vi "Calculate_(101)_Local_Cost_F()-1.vi"(4 "[IN] Dot matrix with statuses \nfor potentially moving dots":i16[][](array[numeric]), 5 "[IN] Still connected\ntracks in group":T1, 6 "[IN] Potentially\nMoving (X,Y)":dbl[][](array[numeric]), 7 "[IN] Subtracks":T2(array[cluster]), 8 "error IN":errorcluster, 9 "[IN] Areas particles\nPrimary Detected":dbl[][](array[numeric]), 10 "[IN] Primary \n(X,Y) Detected":dbl[][](array[numeric]), 11 "[IN] Cost function":i8[](array[numeric])) -> (0 "error OUT":errorcluster, 3 "[OUT] Cost function":i8[](array[numeric]))   [LabVIEW 2013]
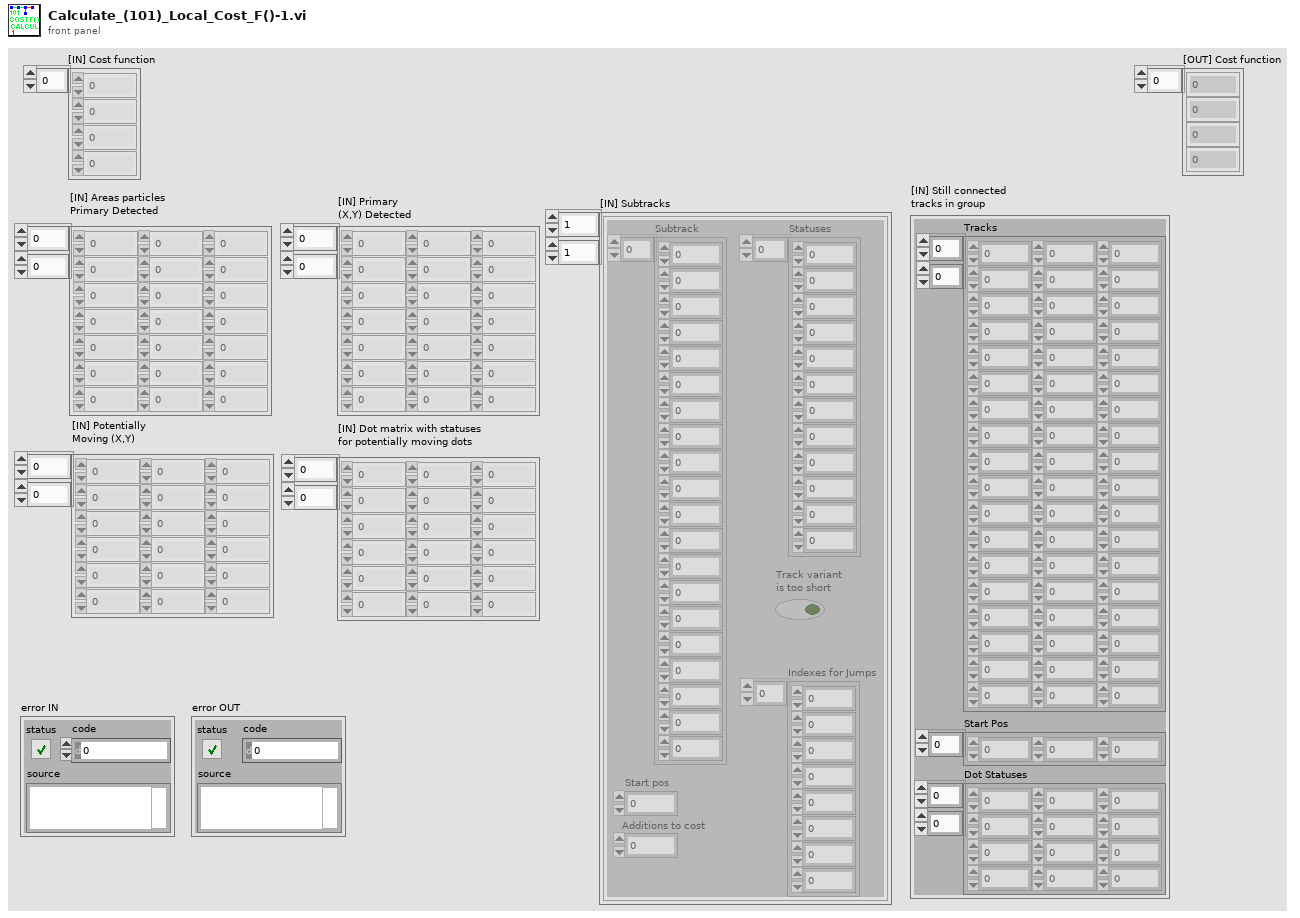
[diagram p1: front panel]
types:
  T1 = cluster{"Tracks":dbl[][], "Start Pos":i32[], "Dot Statuses":i16[][]}
  T2 = cluster{"Subtrack":dbl[], "Statuses":i16[], "Start pos":i32, "Additions to cost":i32, "Track variant \nis too short":bool, "Indexes for Jumps":i32[]}[][]
  T3 = cluster{"Subtrack":dbl[], "Statuses":i16[], "Start pos":i32, "Additions to cost":i32, "Track variant \nis too short":bool, "Indexes for Jumps":i32[]}[]
  T4 = cluster{"Subtrack":dbl[], "Statuses":i16[], "Start pos":i32, "Additions to cost":i32, "Track variant \nis too short":bool, "Indexes for Jumps":i32[]}
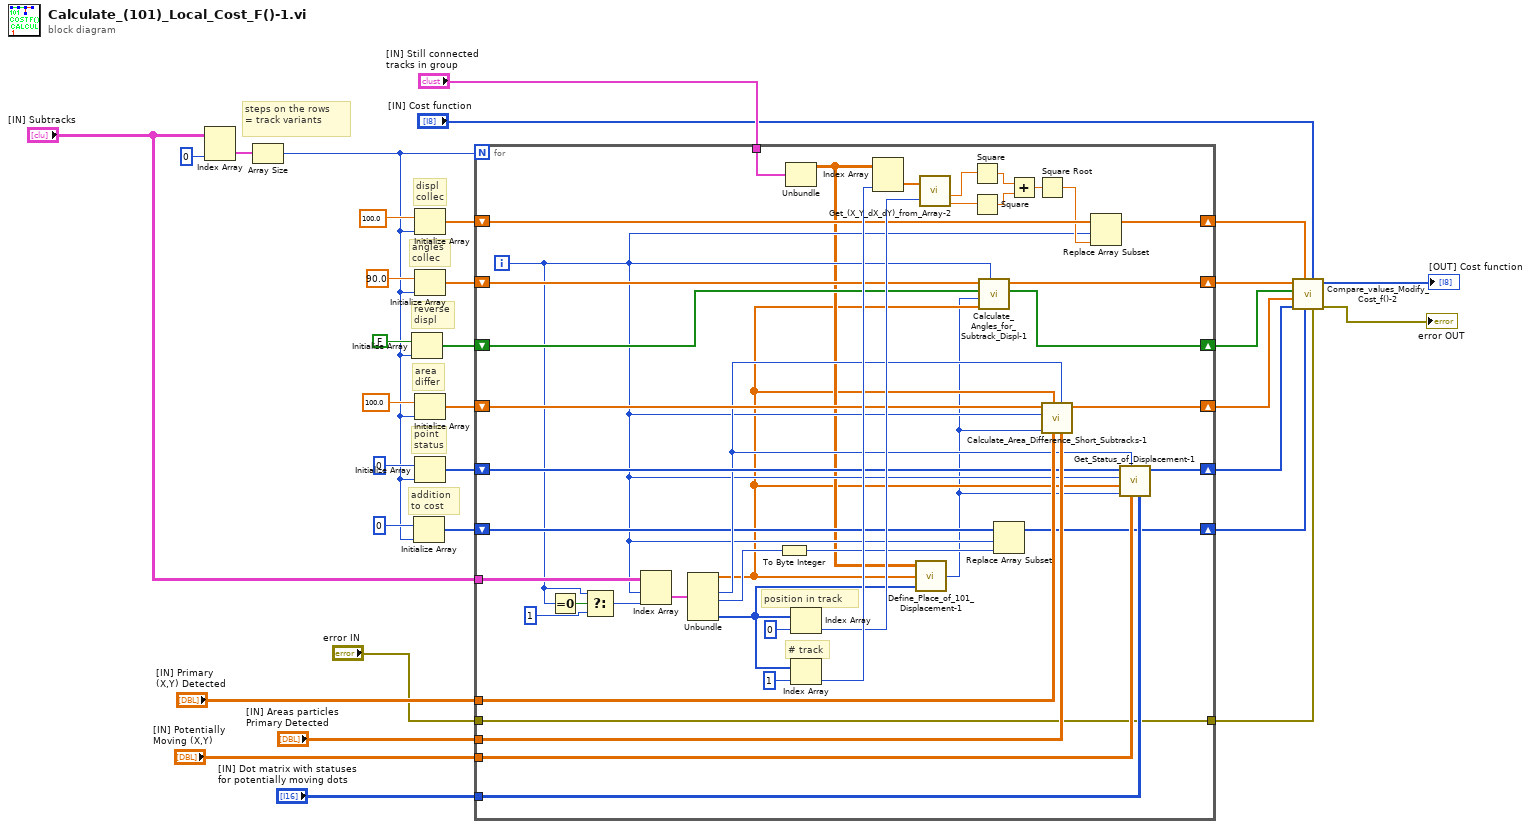
[diagram p0: block diagram]
diagram:
  # "steps on the rows\n= track variants"
  # "addition \nto cost"
  # "point\nstatus"
  # "area \ndiffer"
  # "reverse \ndispl"
  # "angles \ncollec"
  # "displ \ncollec"
  n1 = Index Array(array="[IN] Subtracks", index (col)=0 ("disabled index (col)")) -> (element=w18:T3)  [unwired: 1 in]
  n2 = Array Size(array=w18) -> (size(s)=w17:i32)
  n3 = Initialize Array(FALSE, w17) -> (w27:bool[])
  n4 = Initialize Array(i8 0, w17) -> (w21:i8[])
  n5 = Initialize Array(100.0, w17) -> (w31:dbl[])
  n6 = Initialize Array(90.0, w17) -> (w29:dbl[])
  n7 = Initialize Array(100.0, w17) -> (w25:dbl[])
  n8 = Initialize Array(i16 0, w17) -> (w23:i16[])
  n9 = for {
    N: w17 -> [_]
    tunnel: "[IN] Subtracks" -> [w74]
    tunnel: "[IN] Still connected\ntracks in group" -> [w70]
    shift-right: [w65] -> w6
    shift-left: w31 -> [w66]
    shift-right: [w63] -> w10
    shift-left: w29 -> [w64]
    shift-right: [w61] -> w9
    shift-left: w27 -> [w62]
    tunnel: "[IN] Primary \n(X,Y) Detected" -> [w57]
    tunnel: "[IN] Areas particles\nPrimary Detected" -> [w59]
    shift-right: [w58] -> w8
    shift-left: w25 -> [w60]
    tunnel: "[IN] Potentially\nMoving (X,Y)" -> [w54]
    tunnel: "[IN] Dot matrix with statuses \nfor potentially moving dots" -> [w53]
    shift-right: [w52] -> w7
    shift-left: w23 -> [w56]
    shift-right: [w48] -> w4
    shift-left: w21 -> [w51]
    tunnel: "error IN" -> [w41]
    tunnel: [w41] -> w2
    i -> [w37]
    # "# track"
    # "position in track"
    n10 = Equal To 0?(x=w37) -> (x = 0?=w40:bool)
    n11 = Select(t=w37, s=w40, f=1) -> (s? t:f=w38:i32)
    n12 = Index Array(array=w74, index (row)=w37, index (col)=w38) -> (element=w73:T4)
    n13 = Unbundle(w73) -> ("Subtrack"=w35:dbl[], "Start pos"=w55:i32, "Additions to cost"=w50:i32, "Indexes for Jumps"=w34:i32[])  [unwired: 2 out]
    n14 = To Byte Integer(number=w50) -> (8bit integer=w49:i8)
    n15 = Unbundle(w70) -> ("Tracks"=w36:dbl[][])  [unwired: 2 out]
    n16 = Index Array(array=w34, index=0) -> (element=w67:i32)
    n17 = Index Array(array=w34, index=1) -> (element=w69:i32)
    n18 = Index Array(array=w36, index (col)=w69) -> (element=w68:dbl[])  [unwired: 1 in]
    n19 = call "Define_Place_of_101_Displacement-1.vi"("[IN] Indexes for Jumps"=w34, "[IN] Subtrack"=w35, "[IN] Tracks"=w36) -> ("[OUT] Index of \"11\" Dis\nplacement in Subtrack"=w33:i32)  [unwired: 2 in]
    n20 = call "Get_(X_Y_dX_dY)_from_Array-2.vi"("(X,Y,dX,dY)"=w68, "Index of Displacement"=w67) -> ("dX"=w44:dbl, "dY"=w43:dbl)  [unwired: 2 out]
    n21 = Square(x=w44) -> (x^2=w47:dbl)
    n22 = Square(x=w43) -> (x^2=w46:dbl)
    n23 = call "Calculate_Angles_for_Subtrack_Displ-1.vi"("[IN] Index of subtrack"=w37, "[IN] Subtrack"=w35, "[IN] Index of \"11\" Dis-\nplacement in Subtrack"=w33, "[IN] Reverse Displ or Not"=w62, "[IN] Array with Angles \nBetween Displacement"=w64) -> ("[OUT] Reverse displacement or not"=w61:bool[], "[OUT] Angles betwe\nen two displacements"=w63:dbl[])  [unwired: 3 in]
    n24 = Replace Array Subset(array=w51, new element=w49, index=w37) -> (w48:i8[])
    n25 = Add(x=w47, y=w46) -> (x+y=w45:dbl)
    n26 = Square Root(x=w45) -> (sqrt(x)=w42:dbl)
    n27 = call "Calculate_Area_Difference_Short_Subtracks-1.vi"("[IN] Areas particles\nPrimary Detected"=w59, "[IN] Start pos"=w55, "[IN] Primary \n(X,Y) Detected"=w57, "[IN] Subtrack"=w35, "[IN] Index of \"11\" Dis-\nplacement in Subtrack"=w33, "[IN] Index of\n subtrack"=w37, "[IN] Areas \ndifference"=w60) -> ("[OUT] Areas \ndifference"=w58:dbl[])  [unwired: 4 in]
    n28 = Replace Array Subset(array=w66, new element=w42, index=w37) -> (w65:dbl[])
    n29 = call "Get_Status_of_Displacement-1.vi"("[IN] Dot matrix with statuses\nfor potentially moving dots"=w53, "[IN] Potentially\nMoving (X,Y)"=w54, "[IN] Start pos"=w55, "[IN] Index of Problem\nPoint in Subtrack"=w33, "[IN] Subtrack"=w35, "[IN] Index of\n subtrack"=w37, "[IN] Displace-\nment Statuses"=w56) -> ("[OUT] Displace\nment Statuses"=w52:i16[])  [unwired: 4 in]
  }
  n30 = call "Compare_values_Modify_Cost_f()-2.vi"("error IN"=w2, "[IN] Cost function"="[IN] Cost function", "[IN] Additions to cost"=w4, "[IN] Array of displa\ncement differences"=w6, "[IN] Statuses of points"=w7, "[IN] Areas \ndifferences"=w8, "[IN] Reverse or not"=w9, "[IN] Angles betwe\nen displacements"=w10) -> ("error OUT"=→"error OUT":errorcluster, "[OUT] Cost function"=→"[OUT] Cost function":i8[])  [unwired: 2 in]
